vi "DataFinder Pause or Resume.vi"(8 "error in (no error)":errorcluster, 11 "Action":enum16{"Pause", "Resume"}(ring)) -> (0 "error out":errorcluster)   [LabVIEW 2011]
uses:
  DIAdem/Datasheet/CGI Script Parameters.ctl
  DIAdem/Datasheet/Datasheet Generator Settings.ctl
  server lib/Spartan Version.vi
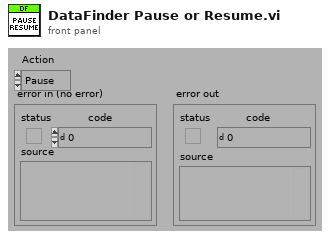
[diagram p1: front panel]
types:
  T1 = typedef "DATASHEET Generator Settings.ctl" = cluster{"Wait? (t)":bool, "ClientPrint? (f)":bool, "Client (\"\")":string, "joinPDF":bool, "Sort Method":enum16{"Item", "Template", "No Sort"}, "Export Row (-1=all)":i32, "Preview":bool, "Estimate Time":bool, "username":string, "jobid":string}
  T2 = typedef "cgi Script parameters.ctl" = cluster{"Report Destination Path":path, "Script":string, "Total Parameters":dbl, "Parameter Names":string[], "Parameter Values":string[], "Scripts":string[], "Run Query?":bool}
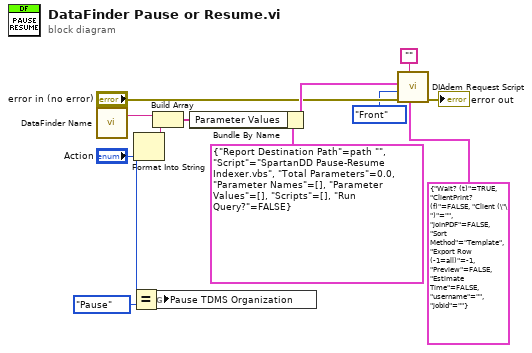
[diagram p0: block diagram]
diagram:
  n1 = call "DataFinder Name.vi"() -> ("DataFinder Name"=w4:string)  [unwired: 3 in]
  n2 = Equal?(x="Action", y=enum16{"Pause", "Resume"}."Pause") -> (x = y?=w1:bool)
  n3 = Format Into String("Action") -> (resulting string=w9:string)  [unwired: 3 in, 1 out]
  n4 = Build Array(w4, w9) -> (w11:string[])
  n5 = global write "Spartan Version.vi" "Pause TDMS Organization"(w1) -> ()
  n6 = Bundle By Name(cluster=T2 {"Report Destination Path"=path "", "Script"="SpartanDD Pause-Resume Indexer.vbs", "Total Parameters"=0.0, "Parameter Names"=[], "Parameter Values"=[], "Scripts"=[], "Run Query?"=FALSE} ("Script Parameters"), "Parameter Values"=w11) -> (w12:T2)
  n7 = call "DIAdem Request Script.vi"("generator settings"=T1 {"Wait? (t)"=TRUE, "ClientPrint? (f)"=FALSE, "Client (\"\")"="", "joinPDF"=FALSE, "Sort Method"=enum."Template", "Export Row (-1=all)"=-1, "Preview"=FALSE, "Estimate Time"=FALSE, "username"="", "jobid"=""}, "RunID"="", "error in (no error)"="error in (no error)", "Queue Entry"=enum16{"Front", "Back"}."Front", "Script Parameters"=w12) -> ("error out"=→"error out":errorcluster)  [unwired: 1 in, 5 out]
